vi "Parse TXT Configuration File.vi"(6 "This VI":refnum<vi>, 8 "error in (no error)":errorcluster, 11 "file path (use dialog)":path=path "D:/GE-Reflective-Memory-Custom-Device-multiple-DMA-transfer-master/GE-Reflective-Memory-Custom-Device-multiple-DMA-transfer-master/Example/A.csv") -> (0 "error out":errorcluster, 3 "DMAs":T1[](array[typedef]))   [LabVIEW 2019, in "RefMem DMA System Explorer.lvlib"]
uses:
  controls/Typedef_DMA Instance.ctl
  controls/Typedef_DMA Block Settings.ctl
  controls/Data Channel Type.ctl
  controls/Typedef_Channel Settings.ctl
  RefMem DMA System Explorer.lvlib
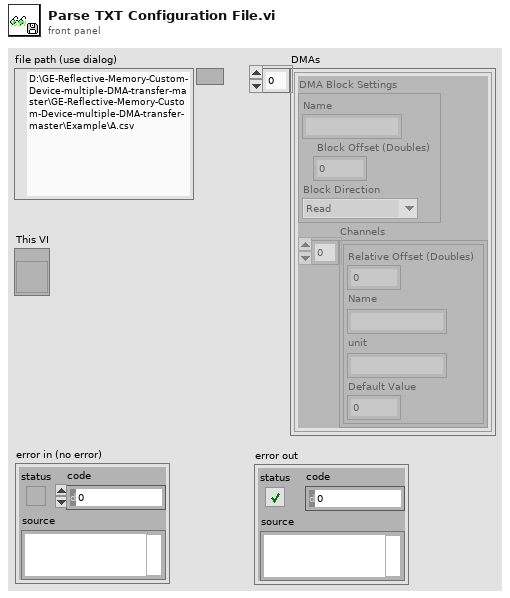
[diagram p1: front panel]
types:
  T1 = typedef "RefMem DMA System Explorer.lvlib/Typedef_DMA Instance.ctl" = cluster{"DMA Block Settings":T2, "Channels":T4[]}
  T2 = typedef "RefMem DMA System Explorer.lvlib/Typedef_DMA Block Settings.ctl" = cluster{"Name":string, " Block Offset (Doubles)":u32, "Block Direction":T3}
  T3 = typedef "RefMem DMA System Explorer.lvlib/Data Channel Type.ctl" = enum16{"Read", "Write"}
  T4 = typedef "RefMem DMA System Explorer.lvlib/Typedef_Channel Settings.ctl" = cluster{"Relative Offset (Doubles)":u32, "Name":string, "unit":string, "Default Value":dbl}
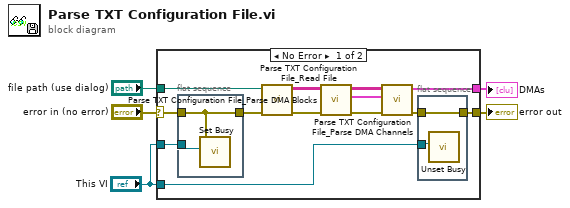
[diagram p0: block diagram]
diagram:
  n1 = case shown="No Error" "error in (no error)" {
    selector: "error in (no error)" -> [w10 w23]
    tunnel: "file path (use dialog)" -> [w18 _]
    tunnel: [w8 w23] -> w4
    tunnel: [w12 _] -> w2
    tunnel: "This VI" -> [w11 _]
    tunnel: "This VI" -> [w7 _]
    frame No Error {
      n2 = flat-sequence {
        tunnel: w11 -> [w20]
        tunnel: w10 -> [w19]
        tunnel: [w19] -> _
        tunnel: [w19] -> w6
        frame #0 {
          n3 = call <vilib>:"Set Busy.vi"("error in (no error)"=w19, "VI reference (current VI)"=w20) -> ()  [unwired: 8 in, 2 out]
        }
      }
      n4 = call "Parse TXT Configuration File_Read File.vi"("error in (no error)"=w6, "file path (use dialog)"=w18) -> ("error out"=w17:errorcluster, "Array"=w13:string[][])  [unwired: 8 in]
      n5 = call "Parse TXT Configuration File_Parse DMA Blocks.vi"("error in (no error)"=w17, "Array in"=w13) -> ("error out"=w14:errorcluster, "DMA Blocks"=w15:T2[], "Array Out"=w16:string[][])  [unwired: 7 in]
      n6 = call "Parse TXT Configuration File_Parse DMA Channels.vi"("error in (no error)"=w14, "DMA Blocks"=w15, "Array in"=w16) -> ("error out"=w9:errorcluster, "DMAs"=w12:T1[])  [unwired: 7 in]
      n7 = flat-sequence {
        tunnel: w9 -> [w22]
        tunnel: [w22] -> w8
        tunnel: w7 -> [w21]
        frame #0 {
          n8 = call <vilib>:"Unset Busy.vi"("VI reference (current VI)"=w21) -> ()  [unwired: 10 in, 1 out]
        }
      }
    }
    frame Error {
    }
  }
  "error out" <- w4
  "DMAs" <- w2
